vi "输入数据解析.vi"(0 "单个参数补充":dbl, 1 "从板号":dbl=1.0, 2 "主板二维码":string="BNET01", 3 "从板二维码":string="BNET01", 5 "主板引用":refnum<vi>, 7 "从板引用":refnum<vi>, 9 "主板选项":string="三级故障阀值", 11 "枚举":enum16{"主板", "从板"}(ring), 12 "快换":bool caption="快换写入") -> (4 "输出数组":dbl[][](array[numeric]), 6 "数组长度":dbl[](array[numeric]), 8 "循环次数":i32, 10 "命令":u32, 14 "名称":string[](array[string]), 15 "命令序号":u32[](array[numeric]))   [LabVIEW 2013] (continued)
                    n4439 = Unbundle By Name(w11573) -> ("总电压过低"=w11572:dbl)
                    n4440 = call "输入分辨率计算-EV05.vi"("1字节?"=FALSE, "数值"=w11572, "分辨率"=0.1) -> ("低字节"=w11575:dbl, "高字节1"=w11574:dbl)  [unwired: 2 in, 5 out]
                  }
                  frame Enabled {
                    w11578 = 255 ("高字节1")
                  }
                }
                n4441 = Build Array(w11570, w11571) -> (w11569:i32[])
              }
              frame 2 {
                # "温度过高"
                n4442 = disable-structure shown="启用" {
                  disable-tunnel: [w11585 255 ("高字节1")] -> w11581
                  disable-tunnel: w11579 -> [w11583 _]
                  frame Disabled {
                    n4443 = Unbundle By Name(w11583) -> ("温度过高"=w11582:dbl)
                    n4444 = call "输入分辨率计算-EV05.vi"("1字节?"=TRUE, "数值"=w11582, "偏移量"=-40.0, "分辨率"=1.0) -> ("高字节1"=w11585:dbl)  [unwired: 1 in, 6 out]
                  }
                  frame Enabled {
                  }
                }
                n4445 = Build Array(w11581) -> (w11580:i32[])
              }
              frame 3 {
                # "温度过低"
                n4446 = disable-structure shown="启用" {
                  disable-tunnel: [w11595 255 ("高字节1")] -> w11591
                  disable-tunnel: w11589 -> [w11593 _]
                  frame Disabled {
                    n4447 = Unbundle By Name(w11593) -> ("温度过低"=w11592:dbl)
                    n4448 = call "输入分辨率计算-EV05.vi"("1字节?"=TRUE, "数值"=w11592, "偏移量"=-40.0, "分辨率"=1.0) -> ("高字节1"=w11595:dbl)  [unwired: 1 in, 6 out]
                  }
                  frame Enabled {
                  }
                }
                n4449 = Build Array(w11591) -> (w11590:i32[])
              }
              frame 4 {
                # "整组温度不均衡"
                n4450 = disable-structure shown="启用" {
                  disable-tunnel: [w11605 255 ("高字节1")] -> w11601
                  disable-tunnel: w11599 -> [w11603 _]
                  frame Disabled {
                    n4451 = Unbundle By Name(w11603) -> ("整组温度不均衡"=w11602:dbl)
                    n4452 = call "输入分辨率计算-EV05.vi"("1字节?"=TRUE, "数值"=w11602, "偏移量"=0.0, "分辨率"=1.0) -> ("高字节1"=w11605:dbl)  [unwired: 1 in, 6 out]
                  }
                  frame Enabled {
                  }
                }
                n4453 = Build Array(w11601) -> (w11600:i32[])
              }
              frame 5 {
                # "单组电压不均衡"
                n4454 = disable-structure shown="启用" {
                  disable-tunnel: [w11617 w11620] -> w11612
                  disable-tunnel: [w11615 w11620] -> w11610
                  disable-tunnel: w11609 -> [w11614 _]
                  frame Disabled {
                    n4455 = Unbundle By Name(w11614) -> ("单组电压不均衡"=w11613:dbl)
                    n4456 = call "输入分辨率计算-EV05.vi"("1字节?"=FALSE, "数值"=w11613, "偏移量"=0.0, "分辨率"=0.001) -> ("低字节"=w11615:dbl, "高字节1"=w11617:dbl)  [unwired: 1 in, 5 out]
                  }
                  frame Enabled {
                    w11620 = 255 ("高字节1")
                  }
                }
                n4457 = Build Array(w11612, w11610) -> (w11611:i32[])
              }
              frame 6 {
                # "整组电压不均衡"
                n4458 = disable-structure shown="启用" {
                  disable-tunnel: [w11629 w11632] -> w11624
                  disable-tunnel: [w11627 w11632] -> w11622
                  disable-tunnel: w11621 -> [w11626 _]
                  frame Disabled {
                    n4459 = Unbundle By Name(w11626) -> ("整组电压不均衡"=w11625:dbl)
                    n4460 = call "输入分辨率计算-EV05.vi"("1字节?"=FALSE, "数值"=w11625, "偏移量"=0.0, "分辨率"=0.001) -> ("低字节"=w11627:dbl, "高字节1"=w11629:dbl)  [unwired: 1 in, 5 out]
                  }
                  frame Enabled {
                    w11632 = 255 ("高字节1")
                  }
                }
                n4461 = Build Array(w11624, w11622) -> (w11623:i32[])
              }
              frame 7 {
                # "单体电压过高"
                n4462 = disable-structure shown="启用" {
                  disable-tunnel: [w11641 w11644] -> w11636
                  disable-tunnel: [w11639 w11644] -> w11634
                  disable-tunnel: w11633 -> [w11638 _]
                  frame Disabled {
                    n4463 = Unbundle By Name(w11638) -> ("单体电压过高"=w11637:dbl)
                    n4464 = call "输入分辨率计算-EV05.vi"("1字节?"=FALSE, "数值"=w11637, "偏移量"=0.0, "分辨率"=0.001) -> ("低字节"=w11639:dbl, "高字节1"=w11641:dbl)  [unwired: 1 in, 5 out]
                  }
                  frame Enabled {
                    w11644 = 255 ("高字节1")
                  }
                }
                n4465 = Build Array(w11636, w11634) -> (w11635:i32[])
              }
              frame 8 {
                # "单体电压过低"
                n4466 = disable-structure shown="启用" {
                  disable-tunnel: [w11653 w11656] -> w11648
                  disable-tunnel: [w11651 w11656] -> w11646
                  disable-tunnel: w11645 -> [w11650 _]
                  frame Disabled {
                    n4467 = Unbundle By Name(w11650) -> ("单体电压过低"=w11649:dbl)
                    n4468 = call "输入分辨率计算-EV05.vi"("1字节?"=FALSE, "数值"=w11649, "偏移量"=0.0, "分辨率"=0.001) -> ("低字节"=w11651:dbl, "高字节1"=w11653:dbl)  [unwired: 1 in, 5 out]
                  }
                  frame Enabled {
                    w11656 = 255 ("高字节1")
                  }
                }
                n4469 = Build Array(w11648, w11646) -> (w11647:i32[])
              }
              frame 9 {
                # "充电电流过高"
                n4470 = disable-structure shown="启用" {
                  disable-tunnel: [w11665 w11668] -> w11660
                  disable-tunnel: [w11663 w11668] -> w11658
                  disable-tunnel: w11657 -> [w11662 _]
                  frame Disabled {
                    n4471 = Unbundle By Name(w11662) -> ("充电电流过高"=w11661:dbl)
                    n4472 = call "输入分辨率计算-EV05.vi"("1字节?"=FALSE, "数值"=w11661, "偏移量"=-3000.0, "分辨率"=0.1) -> ("低字节"=w11663:dbl, "高字节1"=w11665:dbl)  [unwired: 1 in, 5 out]
                  }
                  frame Enabled {
                    w11668 = 255 ("高字节1")
                  }
                }
                n4473 = Build Array(w11660, w11658) -> (w11659:i32[])
              }
              frame 10 {
                # "放电电流过高"
                n4474 = disable-structure shown="启用" {
                  disable-tunnel: [w11677 w11680] -> w11672
                  disable-tunnel: [w11675 w11680] -> w11670
                  disable-tunnel: w11669 -> [w11674 _]
                  frame Disabled {
                    n4475 = Unbundle By Name(w11674) -> ("放电电流过高"=w11673:dbl)
                    n4476 = call "输入分辨率计算-EV05.vi"("1字节?"=FALSE, "数值"=w11673, "偏移量"=-3000.0, "分辨率"=0.1) -> ("低字节"=w11675:dbl, "高字节1"=w11677:dbl)  [unwired: 1 in, 5 out]
                  }
                  frame Enabled {
                    w11680 = 255 ("高字节1")
                  }
                }
                n4477 = Build Array(w11672, w11670) -> (w11671:i32[])
              }
              frame 11 {
                # "单组温度不均衡"
                n4478 = disable-structure shown="启用" {
                  disable-tunnel: [w11687 255 ("高字节1")] -> w11683
                  disable-tunnel: w11681 -> [w11685 _]
                  frame Disabled {
                    n4479 = Unbundle By Name(w11685) -> ("单组温度不均衡"=w11684:dbl)
                    n4480 = call "输入分辨率计算-EV05.vi"("1字节?"=TRUE, "数值"=w11684, "偏移量"=0.0, "分辨率"=1.0) -> ("高字节1"=w11687:dbl)  [unwired: 1 in, 6 out]
                  }
                  frame Enabled {
                  }
                }
                n4481 = Build Array(w11683) -> (w11682:i32[])
              }
              frame 12 {
                # "SOC过高"
                n4482 = Unbundle By Name(w11694) -> ("SOC过高"=w11693:dbl)
                n4483 = call "输入分辨率计算-EV05.vi"("1字节?"=FALSE, "数值"=w11693, "偏移量"=0.0, "分辨率"=0.1) -> ("低字节"=w11691:dbl, "高字节1"=w11692:dbl)  [unwired: 1 in, 5 out]
                n4484 = Build Array(w11692, w11691) -> (w11696:dbl[])
              }
              frame 13 {
                # "SOC过低"
                n4485 = disable-structure shown="启用" {
                  disable-tunnel: w11701 -> [w11706 _]
                  disable-tunnel: [w11704 w11710] -> w11700
                  disable-tunnel: [w11703 w11710] -> w11699
                  frame Disabled {
                    n4486 = Unbundle By Name(w11706) -> ("SOC过低"=w11705:dbl)
                    n4487 = call "输入分辨率计算-EV05.vi"("1字节?"=FALSE, "数值"=w11705, "偏移量"=0.0, "分辨率"=0.1) -> ("低字节"=w11703:dbl, "高字节1"=w11704:dbl)  [unwired: 1 in, 5 out]
                  }
                  frame Enabled {
                    w11710 = 255 ("高字节1")
                  }
                }
                n4488 = Build Array(w11700, w11699) -> (w11702:i32[])
              }
              frame 14 {
                # "内阻过大"
                n4489 = disable-structure shown="启用" {
                  disable-tunnel: w11713 -> [w11718 _]
                  disable-tunnel: [w11714 255 ("高字节1")] -> w11711
                  frame Disabled {
                    n4490 = Unbundle By Name(w11718) -> ("内阻过大"=w11717:dbl)
                    n4491 = call "输入分辨率计算-EV05.vi"("1字节?"=TRUE, "数值"=w11717, "分辨率"=0.1) -> ("高字节1"=w11714:dbl)  [unwired: 2 in, 6 out]
                  }
                  frame Enabled {
                  }
                }
                n4492 = Build Array(w11711) -> (w11712:i32[])
              }
              frame 15 {
                # "极柱温度过高"
                n4493 = disable-structure shown="启用" {
                  disable-tunnel: w11722 -> [w11728 _]
                  disable-tunnel: [w11724 255 ("高字节1")] -> w11720
                  frame Disabled {
                    n4494 = Unbundle By Name(w11728) -> ("极柱温度过高"=w11727:dbl)
                    n4495 = call "输入分辨率计算-EV05.vi"("1字节?"=TRUE, "数值"=w11727, "偏移量"=-40.0, "分辨率"=1.0) -> ("高字节1"=w11724:dbl)  [unwired: 1 in, 6 out]
                  }
                  frame Enabled {
                  }
                }
                n4496 = Build Array(w11720) -> (w11721:i32[])
              }
              frame 16 {
                # "SOH过低"
                n4497 = disable-structure shown="启用" {
                  disable-tunnel: [w11745 w11753] -> w11732
                  disable-tunnel: w11731 -> [w11742 _]
                  disable-tunnel: [w11734 w11753] -> w11730
                  frame Disabled {
                    n4498 = Unbundle By Name(w11742) -> ("SOH过低"=w11741:dbl)
                    n4499 = call "输入分辨率计算-EV05.vi"("1字节?"=FALSE, "数值"=w11741, "偏移量"=0.0, "分辨率"=0.1) -> ("低字节"=w11743:dbl, "高字节1"=w11744:dbl)  [unwired: 1 in, 5 out]
                    n4500 = call "二进制解析-8.6.vi"("索引"=4, "数值"=w11744) -> ("低位子数组"=w11747:i32[])  [unwired: 3 out]
                    n4501 = call "二进制解析-8.6.vi"("索引"=4, "数值"=w11743) -> ("低位子数组"=w11736:i32[], "高位子数组"=w11746:i32[])  [unwired: 2 out]
                    n4502 = call "二进制解析-8.6.vi"("索引"=4, "数值"=0) -> ("低位子数组"=w11737:i32[])  [unwired: 3 out]
                    n4503 = Insert Into Array(array=w11747, new element=w11746) -> (w11740:i32[])  [unwired: 1 in]
                    n4504 = Insert Into Array(array=w11736, new element=w11737) -> (w11735:i32[])  [unwired: 1 in]
                    n4505 = call "数值二进制转十进制-8.6.vi"("子数组"=w11740) -> ("十进制数值"=w11745:i32)  [unwired: 4 out]
                    n4506 = call "数值二进制转十进制-8.6.vi"("子数组"=w11735) -> ("十进制数值"=w11734:i32)  [unwired: 4 out]
                  }
                  frame Enabled {
                    w11753 = 255 ("高字节1")
                  }
                }
                n4507 = Build Array(w11732, w11730) -> (w11733:i32[])
              }
            }
            n4508 = Insert Into Array(array=w11553, new element=w11554) -> (w11552:dbl[])  [unwired: 1 in]
          }
          n4509 = Build Array(w11549) -> (w11548:dbl[][])
          n4510 = Build Array("二级故障阀值") -> (w11539:string[])
        }
        frame "SOC过高(3)" {
          n4511 = Unbundle By Name(w11759) -> ("一级故障 3"=w11760:refnum<vi>)
          n4512 = property class="Clust (严格)"(reference=w11760) -> ("Value"=w11758:T4)  [unwired: 1 in, 2 out]
          n4513 = for {
            N: 17 -> [_]
            tunnel: w11758 -> [w11770]
            shift-right: [w11767] -> w11764
            shift-left: dbl[] [] -> [w11768]
            i -> [w11771]
            n4514 = case shown="12" w11771 {
              tunnel: w11770 -> [w11772 w11783 w11794 w11804 w11814 w11824 w11836 w11848 w11860 w11872 w11884 w11896 w11909 w11917 w11924 w11933 w11942]
              tunnel: [w11773 w11784 w11795 w11805 w11815 w11826 w11838 w11850 w11862 w11874 w11886 w11897 w11911 w11919 w11923 w11932 w11944] -> w11769
              frame 0, Default {
                # "总电压过高"
                n4515 = disable-structure shown="启用" {
                  disable-tunnel: [w11779 w11782] -> w11775
                  disable-tunnel: [w11778 w11782] -> w11774
                  disable-tunnel: w11772 -> [w11777 _]
                  frame Disabled {
                    n4516 = Unbundle By Name(w11777) -> ("总电压过高"=w11776:dbl)
                    n4517 = call "输入分辨率计算-EV05.vi"("1字节?"=FALSE, "数值"=w11776, "分辨率"=0.1) -> ("低字节"=w11779:dbl, "高字节1"=w11778:dbl)  [unwired: 2 in, 5 out]
                  }
                  frame Enabled {
                    w11782 = 255 ("高字节1")
                  }
                }
                n4518 = Build Array(w11774, w11775) -> (w11773:i32[])
              }
              frame 1 {
                # "总电压过低"
                n4519 = disable-structure shown="启用" {
                  disable-tunnel: [w11790 w11793] -> w11786
                  disable-tunnel: [w11789 w11793] -> w11785
                  disable-tunnel: w11783 -> [w11788 _]
                  frame Disabled {
                    n4520 = Unbundle By Name(w11788) -> ("总电压过低"=w11787:dbl)
                    n4521 = call "输入分辨率计算-EV05.vi"("1字节?"=FALSE, "数值"=w11787, "分辨率"=0.1) -> ("低字节"=w11790:dbl, "高字节1"=w11789:dbl)  [unwired: 2 in, 5 out]
                  }
                  frame Enabled {
                    w11793 = 255 ("高字节1")
                  }
                }
                n4522 = Build Array(w11785, w11786) -> (w11784:i32[])
              }
              frame 2 {
                # "温度过高"
                n4523 = disable-structure shown="启用" {
                  disable-tunnel: [w11800 255 ("高字节1")] -> w11796
                  disable-tunnel: w11794 -> [w11798 _]
                  frame Disabled {
                    n4524 = Unbundle By Name(w11798) -> ("温度过高"=w11797:dbl)
                    n4525 = call "输入分辨率计算-EV05.vi"("1字节?"=TRUE, "数值"=w11797, "偏移量"=-40.0, "分辨率"=1.0) -> ("高字节1"=w11800:dbl)  [unwired: 1 in, 6 out]
                  }
                  frame Enabled {
                  }
                }
                n4526 = Build Array(w11796) -> (w11795:i32[])
              }
              frame 3 {
                # "温度过低"
                n4527 = disable-structure shown="启用" {
                  disable-tunnel: [w11810 255 ("高字节1")] -> w11806
                  disable-tunnel: w11804 -> [w11808 _]
                  frame Disabled {
                    n4528 = Unbundle By Name(w11808) -> ("温度过低"=w11807:dbl)
                    n4529 = call "输入分辨率计算-EV05.vi"("1字节?"=TRUE, "数值"=w11807, "偏移量"=-40.0, "分辨率"=1.0) -> ("高字节1"=w11810:dbl)  [unwired: 1 in, 6 out]
                  }
                  frame Enabled {
                  }
                }
                n4530 = Build Array(w11806) -> (w11805:i32[])
              }
              frame 4 {
                # "整组温度不均衡"
                n4531 = disable-structure shown="启用" {
                  disable-tunnel: [w11820 255 ("高字节1")] -> w11816
                  disable-tunnel: w11814 -> [w11818 _]
                  frame Disabled {
                    n4532 = Unbundle By Name(w11818) -> ("整组温度不均衡"=w11817:dbl)
                    n4533 = call "输入分辨率计算-EV05.vi"("1字节?"=TRUE, "数值"=w11817, "偏移量"=0.0, "分辨率"=1.0) -> ("高字节1"=w11820:dbl)  [unwired: 1 in, 6 out]
                  }
                  frame Enabled {
                  }
                }
                n4534 = Build Array(w11816) -> (w11815:i32[])
              }
              frame 5 {
                # "单组电压不均衡"
                n4535 = disable-structure shown="启用" {
                  disable-tunnel: [w11832 w11835] -> w11827
                  disable-tunnel: [w11830 w11835] -> w11825
                  disable-tunnel: w11824 -> [w11829 _]
                  frame Disabled {
                    n4536 = Unbundle By Name(w11829) -> ("单组电压不均衡"=w11828:dbl)
                    n4537 = call "输入分辨率计算-EV05.vi"("1字节?"=FALSE, "数值"=w11828, "偏移量"=0.0, "分辨率"=0.001) -> ("低字节"=w11830:dbl, "高字节1"=w11832:dbl)  [unwired: 1 in, 5 out]
                  }
                  frame Enabled {
                    w11835 = 255 ("高字节1")
                  }
                }
                n4538 = Build Array(w11827, w11825) -> (w11826:i32[])
              }
              frame 6 {
                # "整组电压不均衡"
                n4539 = disable-structure shown="启用" {
                  disable-tunnel: [w11844 w11847] -> w11839
                  disable-tunnel: [w11842 w11847] -> w11837
                  disable-tunnel: w11836 -> [w11841 _]
                  frame Disabled {
                    n4540 = Unbundle By Name(w11841) -> ("整组电压不均衡"=w11840:dbl)
                    n4541 = call "输入分辨率计算-EV05.vi"("1字节?"=FALSE, "数值"=w11840, "偏移量"=0.0, "分辨率"=0.001) -> ("低字节"=w11842:dbl, "高字节1"=w11844:dbl)  [unwired: 1 in, 5 out]
                  }
                  frame Enabled {
                    w11847 = 255 ("高字节1")
                  }
                }
                n4542 = Build Array(w11839, w11837) -> (w11838:i32[])
              }
              frame 7 {
                # "单体电压过高"
                n4543 = disable-structure shown="启用" {
                  disable-tunnel: [w11856 w11859] -> w11851
                  disable-tunnel: [w11854 w11859] -> w11849
                  disable-tunnel: w11848 -> [w11853 _]
                  frame Disabled {
                    n4544 = Unbundle By Name(w11853) -> ("单体电压过高"=w11852:dbl)
                    n4545 = call "输入分辨率计算-EV05.vi"("1字节?"=FALSE, "数值"=w11852, "偏移量"=0.0, "分辨率"=0.001) -> ("低字节"=w11854:dbl, "高字节1"=w11856:dbl)  [unwired: 1 in, 5 out]
                  }
                  frame Enabled {
                    w11859 = 255 ("高字节1")
                  }
                }
                n4546 = Build Array(w11851, w11849) -> (w11850:i32[])
              }
              frame 8 {
                # "单体电压过低"
                n4547 = disable-structure shown="启用" {
                  disable-tunnel: [w11868 w11871] -> w11863
                  disable-tunnel: [w11866 w11871] -> w11861
                  disable-tunnel: w11860 -> [w11865 _]
                  frame Disabled {
                    n4548 = Unbundle By Name(w11865) -> ("单体电压过低"=w11864:dbl)
                    n4549 = call "输入分辨率计算-EV05.vi"("1字节?"=FALSE, "数值"=w11864, "偏移量"=0.0, "分辨率"=0.001) -> ("低字节"=w11866:dbl, "高字节1"=w11868:dbl)  [unwired: 1 in, 5 out]
                  }
                  frame Enabled {
                    w11871 = 255 ("高字节1")
                  }
                }
                n4550 = Build Array(w11863, w11861) -> (w11862:i32[])
              }
              frame 9 {
                # "充电电流过高"
                n4551 = disable-structure shown="启用" {
                  disable-tunnel: [w11880 w11883] -> w11875
                  disable-tunnel: [w11878 w11883] -> w11873
                  disable-tunnel: w11872 -> [w11877 _]
                  frame Disabled {
                    n4552 = Unbundle By Name(w11877) -> ("充电电流过高"=w11876:dbl)
                    n4553 = call "输入分辨率计算-EV05.vi"("1字节?"=FALSE, "数值"=w11876, "偏移量"=-3000.0, "分辨率"=0.1) -> ("低字节"=w11878:dbl, "高字节1"=w11880:dbl)  [unwired: 1 in, 5 out]
                  }
                  frame Enabled {
                    w11883 = 255 ("高字节1")
                  }
                }
                n4554 = Build Array(w11875, w11873) -> (w11874:i32[])
              }
              frame 10 {
                # "放电电流过高"
                n4555 = disable-structure shown="启用" {
                  disable-tunnel: [w11892 w11895] -> w11887
                  disable-tunnel: [w11890 w11895] -> w11885
                  disable-tunnel: w11884 -> [w11889 _]
                  frame Disabled {
                    n4556 = Unbundle By Name(w11889) -> ("放电电流过高"=w11888:dbl)
                    n4557 = call "输入分辨率计算-EV05.vi"("1字节?"=FALSE, "数值"=w11888, "偏移量"=-3000.0, "分辨率"=0.1) -> ("低字节"=w11890:dbl, "高字节1"=w11892:dbl)  [unwired: 1 in, 5 out]
                  }
                  frame Enabled {
                    w11895 = 255 ("高字节1")
                  }
                }
                n4558 = Build Array(w11887, w11885) -> (w11886:i32[])
              }
              frame 11 {
                # "单组温度不均衡"
                n4559 = disable-structure shown="启用" {
                  disable-tunnel: [w11902 255 ("高字节1")] -> w11898
                  disable-tunnel: w11896 -> [w11900 _]
                  frame Disabled {
                    n4560 = Unbundle By Name(w11900) -> ("单组温度不均衡"=w11899:dbl)
                    n4561 = call "输入分辨率计算-EV05.vi"("1字节?"=TRUE, "数值"=w11899, "偏移量"=0.0, "分辨率"=1.0) -> ("高字节1"=w11902:dbl)  [unwired: 1 in, 6 out]
                  }
                  frame Enabled {
                  }
                }
                n4562 = Build Array(w11898) -> (w11897:i32[])
              }
              frame 12 {
                # "SOC过高"
                n4563 = Unbundle By Name(w11909) -> ("SOC过高"=w11908:dbl)
                n4564 = call "输入分辨率计算-EV05.vi"("1字节?"=FALSE, "数值"=w11908, "偏移量"=0.0, "分辨率"=0.1) -> ("低字节"=w11906:dbl, "高字节1"=w11907:dbl)  [unwired: 1 in, 5 out]
                n4565 = Build Array(w11907, w11906) -> (w11911:dbl[])
              }
              frame 13 {
                # "SOC过低"
                n4566 = Unbundle By Name(w11917) -> ("SOC过低"=w11916:dbl)
                n4567 = call "输入分辨率计算-EV05.vi"("1字节?"=FALSE, "数值"=w11916, "偏移量"=0.0, "分辨率"=0.1) -> ("低字节"=w11914:dbl, "高字节1"=w11915:dbl)  [unwired: 1 in, 5 out]
                n4568 = Build Array(w11915, w11914) -> (w11919:dbl[])
              }
              frame 14 {
                # "内阻过大"
                n4569 = disable-structure shown="启用" {
                  disable-tunnel: w11924 -> [w11929 _]
                  disable-tunnel: [w11925 255 ("高字节1")] -> w11922
                  frame Disabled {
                    n4570 = Unbundle By Name(w11929) -> ("内阻过大"=w11928:dbl)
                    n4571 = call "输入分辨率计算-EV05.vi"("1字节?"=TRUE, "数值"=w11928, "分辨率"=0.1) -> ("高字节1"=w11925:dbl)  [unwired: 2 in, 6 out]
                  }
                  frame Enabled {
                  }
                }
                n4572 = Build Array(w11922) -> (w11923:i32[])
              }
              frame 15 {
                # "极柱温度过高"
                n4573 = disable-structure shown="启用" {
                  disable-tunnel: w11933 -> [w11939 _]
                  disable-tunnel: [w11935 255 ("高字节1")] -> w11931
                  frame Disabled {
                    n4574 = Unbundle By Name(w11939) -> ("极柱温度过高"=w11938:dbl)
                    n4575 = call "输入分辨率计算-EV05.vi"("1字节?"=TRUE, "数值"=w11938, "偏移量"=-40.0, "分辨率"=1.0) -> ("高字节1"=w11935:dbl)  [unwired: 1 in, 6 out]
                  }
                  frame Enabled {
                  }
                }
                n4576 = Build Array(w11931) -> (w11932:i32[])
              }
              frame 16 {
                # "SOH过低"
                n4577 = disable-structure shown="启用" {
                  disable-tunnel: [w11956 w11964] -> w11943
                  disable-tunnel: w11942 -> [w11953 _]
                  disable-tunnel: [w11945 w11964] -> w11941
                  frame Disabled {
                    n4578 = Unbundle By Name(w11953) -> ("SOH过低"=w11952:dbl)
                    n4579 = call "输入分辨率计算-EV05.vi"("1字节?"=FALSE, "数值"=w11952, "偏移量"=0.0, "分辨率"=0.1) -> ("低字节"=w11954:dbl, "高字节1"=w11955:dbl)  [unwired: 1 in, 5 out]
                    n4580 = call "二进制解析-8.6.vi"("索引"=4, "数值"=w11955) -> ("低位子数组"=w11958:i32[])  [unwired: 3 out]
                    n4581 = call "二进制解析-8.6.vi"("索引"=4, "数值"=w11954) -> ("低位子数组"=w11947:i32[], "高位子数组"=w11957:i32[])  [unwired: 2 out]
                    n4582 = call "二进制解析-8.6.vi"("索引"=4, "数值"=0) -> ("低位子数组"=w11948:i32[])  [unwired: 3 out]
                    n4583 = Insert Into Array(array=w11958, new element=w11957) -> (w11951:i32[])  [unwired: 1 in]
                    n4584 = Insert Into Array(array=w11947, new element=w11948) -> (w11946:i32[])  [unwired: 1 in]
                    n4585 = call "数值二进制转十进制-8.6.vi"("子数组"=w11951) -> ("十进制数值"=w11956:i32)  [unwired: 4 out]
                    n4586 = call "数值二进制转十进制-8.6.vi"("子数组"=w11946) -> ("十进制数值"=w11945:i32)  [unwired: 4 out]
                  }
                  frame Enabled {
                    w11964 = 255 ("高字节1")
                  }
                }
                n4587 = Build Array(w11943, w11941) -> (w11944:i32[])
              }
            }
            n4588 = Insert Into Array(array=w11768, new element=w11769) -> (w11767:dbl[])  [unwired: 1 in]
          }
          n4589 = Build Array(w11764) -> (w11763:dbl[][])
          n4590 = Build Array("三级故障阀值") -> (w11754:string[])
        }
        frame "SOC过低" {
          n4591 = Unbundle By Name(w11970) -> ("一级故障"=w11971:refnum<vi>)
          n4592 = property class="Clust (严格)"(reference=w11971) -> ("Value"=w11969:T4)  [unwired: 1 in, 2 out]
          n4593 = for {
            N: 17 -> [_]
            tunnel: w11969 -> [w11981]
            shift-right: [w11978] -> w11975
            shift-left: dbl[] [] -> [w11979]
            i -> [w11982]
            n4594 = case shown="12" w11982 {
              tunnel: w11981 -> [w11983 w11994 w12005 w12015 w12025 w12035 w12047 w12059 w12071 w12083 w12095 w12107 w12119 w12131 w12138 w12147 w12156]
              tunnel: [w11984 w11995 w12006 w12016 w12026 w12037 w12049 w12061 w12073 w12085 w12097 w12108 w12121 w12133 w12137 w12146 w12158] -> w11980
              frame 0, Default {
                # "总电压过高"
                n4595 = disable-structure shown="启用" {
                  disable-tunnel: [w11990 w11993] -> w11986
                  disable-tunnel: [w11989 w11993] -> w11985
                  disable-tunnel: w11983 -> [w11988 _]
                  frame Disabled {
                    n4596 = Unbundle By Name(w11988) -> ("总电压过高"=w11987:dbl)
                    n4597 = call "输入分辨率计算-EV05.vi"("1字节?"=FALSE, "数值"=w11987, "分辨率"=0.1) -> ("低字节"=w11990:dbl, "高字节1"=w11989:dbl)  [unwired: 2 in, 5 out]
                  }
                  frame Enabled {
                    w11993 = 255 ("高字节1")
                  }
                }
                n4598 = Build Array(w11985, w11986) -> (w11984:i32[])
              }
              frame 1 {
                # "总电压过低"
                n4599 = disable-structure shown="启用" {
                  disable-tunnel: [w12001 w12004] -> w11997
                  disable-tunnel: [w12000 w12004] -> w11996
                  disable-tunnel: w11994 -> [w11999 _]
                  frame Disabled {
                    n4600 = Unbundle By Name(w11999) -> ("总电压过低"=w11998:dbl)
                    n4601 = call "输入分辨率计算-EV05.vi"("1字节?"=FALSE, "数值"=w11998, "分辨率"=0.1) -> ("低字节"=w12001:dbl, "高字节1"=w12000:dbl)  [unwired: 2 in, 5 out]
                  }
                  frame Enabled {
                    w12004 = 255 ("高字节1")
                  }
                }
                n4602 = Build Array(w11996, w11997) -> (w11995:i32[])
              }
              frame 2 {
                # "温度过高"
                n4603 = disable-structure shown="启用" {
                  disable-tunnel: [w12011 255 ("高字节1")] -> w12007
                  disable-tunnel: w12005 -> [w12009 _]
                  frame Disabled {
                    n4604 = Unbundle By Name(w12009) -> ("温度过高"=w12008:dbl)
                    n4605 = call "输入分辨率计算-EV05.vi"("1字节?"=TRUE, "数值"=w12008, "偏移量"=-40.0, "分辨率"=1.0) -> ("高字节1"=w12011:dbl)  [unwired: 1 in, 6 out]
                  }
                  frame Enabled {
                  }
                }
                n4606 = Build Array(w12007) -> (w12006:i32[])
              }
              frame 3 {
                # "温度过低"
                n4607 = disable-structure shown="启用" {
                  disable-tunnel: [w12021 255 ("高字节1")] -> w12017
                  disable-tunnel: w12015 -> [w12019 _]
                  frame Disabled {
                    n4608 = Unbundle By Name(w12019) -> ("温度过低"=w12018:dbl)
                    n4609 = call "输入分辨率计算-EV05.vi"("1字节?"=TRUE, "数值"=w12018, "偏移量"=-40.0, "分辨率"=1.0) -> ("高字节1"=w12021:dbl)  [unwired: 1 in, 6 out]
                  }
                  frame Enabled {
                  }
                }
                n4610 = Build Array(w12017) -> (w12016:i32[])
              }
              frame 4 {
                # "整组温度不均衡"
                n4611 = disable-structure shown="启用" {
                  disable-tunnel: [w12031 255 ("高字节1")] -> w12027
                  disable-tunnel: w12025 -> [w12029 _]
                  frame Disabled {
                    n4612 = Unbundle By Name(w12029) -> ("整组温度不均衡"=w12028:dbl)
                    n4613 = call "输入分辨率计算-EV05.vi"("1字节?"=TRUE, "数值"=w12028, "偏移量"=0.0, "分辨率"=1.0) -> ("高字节1"=w12031:dbl)  [unwired: 1 in, 6 out]
                  }
                  frame Enabled {
                  }
                }
                n4614 = Build Array(w12027) -> (w12026:i32[])
              }
              frame 5 {
                # "单组电压不均衡"
                n4615 = disable-structure shown="启用" {
                  disable-tunnel: [w12043 w12046] -> w12038
                  disable-tunnel: [w12041 w12046] -> w12036
                  disable-tunnel: w12035 -> [w12040 _]
                  frame Disabled {
                    n4616 = Unbundle By Name(w12040) -> ("单组电压不均衡"=w12039:dbl)
                    n4617 = call "输入分辨率计算-EV05.vi"("1字节?"=FALSE, "数值"=w12039, "偏移量"=0.0, "分辨率"=0.001) -> ("低字节"=w12041:dbl, "高字节1"=w12043:dbl)  [unwired: 1 in, 5 out]
                  }
                  frame Enabled {
                    w12046 = 255 ("高字节1")
                  }
                }
                n4618 = Build Array(w12038, w12036) -> (w12037:i32[])
              }
              frame 6 {
                # "整组电压不均衡"
                n4619 = disable-structure shown="启用" {
                  disable-tunnel: [w12055 w12058] -> w12050
                  disable-tunnel: [w12053 w12058] -> w12048
                  disable-tunnel: w12047 -> [w12052 _]
                  frame Disabled {
                    n4620 = Unbundle By Name(w12052) -> ("整组电压不均衡"=w12051:dbl)
                    n4621 = call "输入分辨率计算-EV05.vi"("1字节?"=FALSE, "数值"=w12051, "偏移量"=0.0, "分辨率"=0.001) -> ("低字节"=w12053:dbl, "高字节1"=w12055:dbl)  [unwired: 1 in, 5 out]
                  }
                  frame Enabled {
                    w12058 = 255 ("高字节1")
                  }
                }
                n4622 = Build Array(w12050, w12048) -> (w12049:i32[])
              }
              frame 7 {
                # "单体电压过高"
                n4623 = disable-structure shown="启用" {
                  disable-tunnel: [w12067 w12070] -> w12062
                  disable-tunnel: [w12065 w12070] -> w12060
                  disable-tunnel: w12059 -> [w12064 _]
                  frame Disabled {
                    n4624 = Unbundle By Name(w12064) -> ("单体电压过高"=w12063:dbl)
                    n4625 = call "输入分辨率计算-EV05.vi"("1字节?"=FALSE, "数值"=w12063, "偏移量"=0.0, "分辨率"=0.001) -> ("低字节"=w12065:dbl, "高字节1"=w12067:dbl)  [unwired: 1 in, 5 out]
                  }
                  frame Enabled {
                    w12070 = 255 ("高字节1")
                  }
                }
                n4626 = Build Array(w12062, w12060) -> (w12061:i32[])
              }
              frame 8 {
                # "单体电压过低"
                n4627 = disable-structure shown="启用" {
                  disable-tunnel: [w12079 w12082] -> w12074
                  disable-tunnel: [w12077 w12082] -> w12072
                  disable-tunnel: w12071 -> [w12076 _]
                  frame Disabled {
                    n4628 = Unbundle By Name(w12076) -> ("单体电压过低"=w12075:dbl)
                    n4629 = call "输入分辨率计算-EV05.vi"("1字节?"=FALSE, "数值"=w12075, "偏移量"=0.0, "分辨率"=0.001) -> ("低字节"=w12077:dbl, "高字节1"=w12079:dbl)  [unwired: 1 in, 5 out]
                  }
                  frame Enabled {
                    w12082 = 255 ("高字节1")
                  }
                }
                n4630 = Build Array(w12074, w12072) -> (w12073:i32[])
              }
              frame 9 {
                # "充电电流过高"
                n4631 = disable-structure shown="启用" {
                  disable-tunnel: [w12091 w12094] -> w12086
                  disable-tunnel: [w12089 w12094] -> w12084
                  disable-tunnel: w12083 -> [w12088 _]
                  frame Disabled {
                    n4632 = Unbundle By Name(w12088) -> ("充电电流过高"=w12087:dbl)
                    n4633 = call "输入分辨率计算-EV05.vi"("1字节?"=FALSE, "数值"=w12087, "偏移量"=-3000.0, "分辨率"=0.1) -> ("低字节"=w12089:dbl, "高字节1"=w12091:dbl)  [unwired: 1 in, 5 out]
                  }
                  frame Enabled {
                    w12094 = 255 ("高字节1")
                  }
                }
                n4634 = Build Array(w12086, w12084) -> (w12085:i32[])
              }
              frame 10 {
                # "放电电流过高"
                n4635 = disable-structure shown="启用" {
                  disable-tunnel: [w12103 w12106] -> w12098
                  disable-tunnel: [w12101 w12106] -> w12096
                  disable-tunnel: w12095 -> [w12100 _]
                  frame Disabled {
                    n4636 = Unbundle By Name(w12100) -> ("放电电流过高"=w12099:dbl)
                    n4637 = call "输入分辨率计算-EV05.vi"("1字节?"=FALSE, "数值"=w12099, "偏移量"=-3000.0, "分辨率"=0.1) -> ("低字节"=w12101:dbl, "高字节1"=w12103:dbl)  [unwired: 1 in, 5 out]
                  }
                  frame Enabled {
                    w12106 = 255 ("高字节1")
                  }
                }
                n4638 = Build Array(w12098, w12096) -> (w12097:i32[])
              }
              frame 11 {
                # "单组温度不均衡"
                n4639 = disable-structure shown="启用" {
                  disable-tunnel: [w12113 255 ("高字节1")] -> w12109
                  disable-tunnel: w12107 -> [w12111 _]
                  frame Disabled {
                    n4640 = Unbundle By Name(w12111) -> ("单组温度不均衡"=w12110:dbl)
                    n4641 = call "输入分辨率计算-EV05.vi"("1字节?"=TRUE, "数值"=w12110, "偏移量"=0.0, "分辨率"=1.0) -> ("高字节1"=w12113:dbl)  [unwired: 1 in, 6 out]
                  }
                  frame Enabled {
                  }
                }
                n4642 = Build Array(w12109) -> (w12108:i32[])
              }
              frame 12 {
                # "SOC过高"
                n4643 = Unbundle By Name(w12119) -> ("SOC过高"=w12118:dbl)
                n4644 = call "输入分辨率计算-EV05.vi"("1字节?"=FALSE, "数值"=w12118, "偏移量"=0.0, "分辨率"=0.1) -> ()  [unwired: 1 in, 7 out]
                n4645 = disable-structure shown="启用" {
                  disable-tunnel: _ -> [w12125 _]
                  disable-tunnel: [w12125 255 ("高字节1")] -> w12117
                  disable-tunnel: [w12124 i32[] [] ("低位子数组")] -> _
                  disable-tunnel: _ -> [w12124 _]
                  frame Disabled {
                  }
                  frame Enabled {
                  }
                }
                n4646 = Build Array(w12117, w12117) -> (w12121:i32[])
              }
              frame 13 {
                # "SOC过低"
                n4647 = Unbundle By Name(w12131) -> ("SOC过低"=w12130:dbl)
                n4648 = call "输入分辨率计算-EV05.vi"("1字节?"=FALSE, "数值"=w12130, "偏移量"=0.0, "分辨率"=0.1) -> ("低字节"=w12128:dbl, "高字节1"=w12129:dbl)  [unwired: 1 in, 5 out]
                n4649 = Build Array(w12129, w12128) -> (w12133:dbl[])
              }
              frame 14 {
                # "内阻过大"
                n4650 = disable-structure shown="启用" {
                  disable-tunnel: w12138 -> [w12143 _]
                  disable-tunnel: [w12139 255 ("高字节1")] -> w12136
                  frame Disabled {
                    n4651 = Unbundle By Name(w12143) -> ("内阻过大"=w12142:dbl)
                    n4652 = call "输入分辨率计算-EV05.vi"("1字节?"=TRUE, "数值"=w12142, "分辨率"=0.1) -> ("高字节1"=w12139:dbl)  [unwired: 2 in, 6 out]
                  }
                  frame Enabled {
                  }
                }
                n4653 = Build Array(w12136) -> (w12137:i32[])
              }
              frame 15 {
                # "极柱温度过高"
                n4654 = disable-structure shown="启用" {
                  disable-tunnel: w12147 -> [w12153 _]
                  disable-tunnel: [w12149 255 ("高字节1")] -> w12145
                  frame Disabled {
                    n4655 = Unbundle By Name(w12153) -> ("极柱温度过高"=w12152:dbl)
                    n4656 = call "输入分辨率计算-EV05.vi"("1字节?"=TRUE, "数值"=w12152, "偏移量"=-40.0, "分辨率"=1.0) -> ("高字节1"=w12149:dbl)  [unwired: 1 in, 6 out]
                  }
                  frame Enabled {
                  }
                }
                n4657 = Build Array(w12145) -> (w12146:i32[])
              }
              frame 16 {
                # "SOH过低"
                n4658 = disable-structure shown="启用" {
                  disable-tunnel: [w12170 w12178] -> w12157
                  disable-tunnel: w12156 -> [w12167 _]
                  disable-tunnel: [w12159 w12178] -> w12155
                  frame Disabled {
                    n4659 = Unbundle By Name(w12167) -> ("SOH过低"=w12166:dbl)
                    n4660 = call "输入分辨率计算-EV05.vi"("1字节?"=FALSE, "数值"=w12166, "偏移量"=0.0, "分辨率"=0.1) -> ("低字节"=w12168:dbl, "高字节1"=w12169:dbl)  [unwired: 1 in, 5 out]
                    n4661 = call "二进制解析-8.6.vi"("索引"=4, "数值"=w12169) -> ("低位子数组"=w12172:i32[])  [unwired: 3 out]
                    n4662 = call "二进制解析-8.6.vi"("索引"=4, "数值"=w12168) -> ("低位子数组"=w12161:i32[], "高位子数组"=w12171:i32[])  [unwired: 2 out]
                    n4663 = call "二进制解析-8.6.vi"("索引"=4, "数值"=0) -> ("低位子数组"=w12162:i32[])  [unwired: 3 out]
                    n4664 = Insert Into Array(array=w12172, new element=w12171) -> (w12165:i32[])  [unwired: 1 in]
                    n4665 = Insert Into Array(array=w12161, new element=w12162) -> (w12160:i32[])  [unwired: 1 in]
                    n4666 = call "数值二进制转十进制-8.6.vi"("子数组"=w12165) -> ("十进制数值"=w12170:i32)  [unwired: 4 out]
                    n4667 = call "数值二进制转十进制-8.6.vi"("子数组"=w12160) -> ("十进制数值"=w12159:i32)  [unwired: 4 out]
                  }
                  frame Enabled {
                    w12178 = 255 ("高字节1")
                  }
                }
                n4668 = Build Array(w12157, w12155) -> (w12158:i32[])
              }
            }
            n4669 = Insert Into Array(array=w11979, new element=w11980) -> (w11978:dbl[])  [unwired: 1 in]
          }
          n4670 = Build Array(w11975) -> (w11974:dbl[][])
          n4671 = Build Array("一级故障阀值") -> (w11965:string[])
        }
        frame "SOC过低(2)" {
          n4672 = Unbundle By Name(w12184) -> ("一级故障 2"=w12185:refnum<vi>)
          n4673 = property class="Clust (严格)"(reference=w12185) -> ("Value"=w12183:T4)  [unwired: 1 in, 2 out]
          n4674 = for {
            N: 17 -> [_]
            tunnel: w12183 -> [w12195]
            shift-right: [w12192] -> w12189
            shift-left: dbl[] [] -> [w12193]
            i -> [w12196]
            n4675 = case shown="12" w12196 {
              tunnel: w12195 -> [w12197 w12208 w12219 w12229 w12239 w12249 w12261 w12273 w12285 w12297 w12309 w12321 w12333 w12345 w12352 w12361 w12370]
              tunnel: [w12198 w12209 w12220 w12230 w12240 w12251 w12263 w12275 w12287 w12299 w12311 w12322 w12335 w12347 w12351 w12360 w12372] -> w12194
              frame 0, Default {
                # "总电压过高"
                n4676 = disable-structure shown="启用" {
                  disable-tunnel: [w12204 w12207] -> w12200
                  disable-tunnel: [w12203 w12207] -> w12199
                  disable-tunnel: w12197 -> [w12202 _]
                  frame Disabled {
                    n4677 = Unbundle By Name(w12202) -> ("总电压过高"=w12201:dbl)
                    n4678 = call "输入分辨率计算-EV05.vi"("1字节?"=FALSE, "数值"=w12201, "分辨率"=0.1) -> ("低字节"=w12204:dbl, "高字节1"=w12203:dbl)  [unwired: 2 in, 5 out]
                  }
                  frame Enabled {
                    w12207 = 255 ("高字节1")
                  }
                }
                n4679 = Build Array(w12199, w12200) -> (w12198:i32[])
              }
              frame 1 {
                # "总电压过低"
                n4680 = disable-structure shown="启用" {
                  disable-tunnel: [w12215 w12218] -> w12211
                  disable-tunnel: [w12214 w12218] -> w12210
                  disable-tunnel: w12208 -> [w12213 _]
                  frame Disabled {
                    n4681 = Unbundle By Name(w12213) -> ("总电压过低"=w12212:dbl)
                    n4682 = call "输入分辨率计算-EV05.vi"("1字节?"=FALSE, "数值"=w12212, "分辨率"=0.1) -> ("低字节"=w12215:dbl, "高字节1"=w12214:dbl)  [unwired: 2 in, 5 out]
                  }
                  frame Enabled {
                    w12218 = 255 ("高字节1")
                  }
                }
                n4683 = Build Array(w12210, w12211) -> (w12209:i32[])
              }
              frame 2 {
                # "温度过高"
                n4684 = disable-structure shown="启用" {
                  disable-tunnel: [w12225 255 ("高字节1")] -> w12221
                  disable-tunnel: w12219 -> [w12223 _]
                  frame Disabled {
                    n4685 = Unbundle By Name(w12223) -> ("温度过高"=w12222:dbl)
                    n4686 = call "输入分辨率计算-EV05.vi"("1字节?"=TRUE, "数值"=w12222, "偏移量"=-40.0, "分辨率"=1.0) -> ("高字节1"=w12225:dbl)  [unwired: 1 in, 6 out]
                  }
                  frame Enabled {
                  }
                }
                n4687 = Build Array(w12221) -> (w12220:i32[])
              }
              frame 3 {
                # "温度过低"
                n4688 = disable-structure shown="启用" {
                  disable-tunnel: [w12235 255 ("高字节1")] -> w12231
                  disable-tunnel: w12229 -> [w12233 _]
                  frame Disabled {
                    n4689 = Unbundle By Name(w12233) -> ("温度过低"=w12232:dbl)
                    n4690 = call "输入分辨率计算-EV05.vi"("1字节?"=TRUE, "数值"=w12232, "偏移量"=-40.0, "分辨率"=1.0) -> ("高字节1"=w12235:dbl)  [unwired: 1 in, 6 out]
                  }
                  frame Enabled {
                  }
                }
                n4691 = Build Array(w12231) -> (w12230:i32[])
              }
              frame 4 {
                # "整组温度不均衡"
                n4692 = disable-structure shown="启用" {
                  disable-tunnel: [w12245 255 ("高字节1")] -> w12241
                  disable-tunnel: w12239 -> [w12243 _]
                  frame Disabled {
                    n4693 = Unbundle By Name(w12243) -> ("整组温度不均衡"=w12242:dbl)
                    n4694 = call "输入分辨率计算-EV05.vi"("1字节?"=TRUE, "数值"=w12242, "偏移量"=0.0, "分辨率"=1.0) -> ("高字节1"=w12245:dbl)  [unwired: 1 in, 6 out]
                  }
                  frame Enabled {
                  }
                }
                n4695 = Build Array(w12241) -> (w12240:i32[])
              }
              frame 5 {
                # "单组电压不均衡"
                n4696 = disable-structure shown="启用" {
                  disable-tunnel: [w12257 w12260] -> w12252
                  disable-tunnel: [w12255 w12260] -> w12250
                  disable-tunnel: w12249 -> [w12254 _]
                  frame Disabled {
                    n4697 = Unbundle By Name(w12254) -> ("单组电压不均衡"=w12253:dbl)
                    n4698 = call "输入分辨率计算-EV05.vi"("1字节?"=FALSE, "数值"=w12253, "偏移量"=0.0, "分辨率"=0.001) -> ("低字节"=w12255:dbl, "高字节1"=w12257:dbl)  [unwired: 1 in, 5 out]
                  }
                  frame Enabled {
                    w12260 = 255 ("高字节1")
                  }
                }
                n4699 = Build Array(w12252, w12250) -> (w12251:i32[])
              }
              frame 6 {
                # "整组电压不均衡"
                n4700 = disable-structure shown="启用" {
                  disable-tunnel: [w12269 w12272] -> w12264
                  disable-tunnel: [w12267 w12272] -> w12262
                  disable-tunnel: w12261 -> [w12266 _]
                  frame Disabled {
                    n4701 = Unbundle By Name(w12266) -> ("整组电压不均衡"=w12265:dbl)
                    n4702 = call "输入分辨率计算-EV05.vi"("1字节?"=FALSE, "数值"=w12265, "偏移量"=0.0, "分辨率"=0.001) -> ("低字节"=w12267:dbl, "高字节1"=w12269:dbl)  [unwired: 1 in, 5 out]
                  }
                  frame Enabled {
                    w12272 = 255 ("高字节1")
                  }
                }
                n4703 = Build Array(w12264, w12262) -> (w12263:i32[])
              }
              frame 7 {
                # "单体电压过高"
                n4704 = disable-structure shown="启用" {
                  disable-tunnel: [w12281 w12284] -> w12276
                  disable-tunnel: [w12279 w12284] -> w12274
                  disable-tunnel: w12273 -> [w12278 _]
                  frame Disabled {
                    n4705 = Unbundle By Name(w12278) -> ("单体电压过高"=w12277:dbl)
                    n4706 = call "输入分辨率计算-EV05.vi"("1字节?"=FALSE, "数值"=w12277, "偏移量"=0.0, "分辨率"=0.001) -> ("低字节"=w12279:dbl, "高字节1"=w12281:dbl)  [unwired: 1 in, 5 out]
                  }
                  frame Enabled {
                    w12284 = 255 ("高字节1")
                  }
                }
                n4707 = Build Array(w12276, w12274) -> (w12275:i32[])
              }
              frame 8 {
                # "单体电压过低"
                n4708 = disable-structure shown="启用" {
                  disable-tunnel: [w12293 w12296] -> w12288
                  disable-tunnel: [w12291 w12296] -> w12286
                  disable-tunnel: w12285 -> [w12290 _]
                  frame Disabled {
                    n4709 = Unbundle By Name(w12290) -> ("单体电压过低"=w12289:dbl)
                    n4710 = call "输入分辨率计算-EV05.vi"("1字节?"=FALSE, "数值"=w12289, "偏移量"=0.0, "分辨率"=0.001) -> ("低字节"=w12291:dbl, "高字节1"=w12293:dbl)  [unwired: 1 in, 5 out]
                  }
                  frame Enabled {
                    w12296 = 255 ("高字节1")
                  }
                }
                n4711 = Build Array(w12288, w12286) -> (w12287:i32[])
              }
              frame 9 {
                # "充电电流过高"
                n4712 = disable-structure shown="启用" {
                  disable-tunnel: [w12305 w12308] -> w12300
                  disable-tunnel: [w12303 w12308] -> w12298
                  disable-tunnel: w12297 -> [w12302 _]
                  frame Disabled {
                    n4713 = Unbundle By Name(w12302) -> ("充电电流过高"=w12301:dbl)
                    n4714 = call "输入分辨率计算-EV05.vi"("1字节?"=FALSE, "数值"=w12301, "偏移量"=-3000.0, "分辨率"=0.1) -> ("低字节"=w12303:dbl, "高字节1"=w12305:dbl)  [unwired: 1 in, 5 out]
                  }
                  frame Enabled {
                    w12308 = 255 ("高字节1")
                  }
                }
                n4715 = Build Array(w12300, w12298) -> (w12299:i32[])
              }
              frame 10 {
                # "放电电流过高"
                n4716 = disable-structure shown="启用" {
                  disable-tunnel: [w12317 w12320] -> w12312
                  disable-tunnel: [w12315 w12320] -> w12310
                  disable-tunnel: w12309 -> [w12314 _]
                  frame Disabled {
                    n4717 = Unbundle By Name(w12314) -> ("放电电流过高"=w12313:dbl)
                    n4718 = call "输入分辨率计算-EV05.vi"("1字节?"=FALSE, "数值"=w12313, "偏移量"=-3000.0, "分辨率"=0.1) -> ("低字节"=w12315:dbl, "高字节1"=w12317:dbl)  [unwired: 1 in, 5 out]
                  }
                  frame Enabled {
                    w12320 = 255 ("高字节1")
                  }
                }
                n4719 = Build Array(w12312, w12310) -> (w12311:i32[])
              }
              frame 11 {
                # "单组温度不均衡"
                n4720 = disable-structure shown="启用" {
                  disable-tunnel: [w12327 255 ("高字节1")] -> w12323
                  disable-tunnel: w12321 -> [w12325 _]
                  frame Disabled {
                    n4721 = Unbundle By Name(w12325) -> ("单组温度不均衡"=w12324:dbl)
                    n4722 = call "输入分辨率计算-EV05.vi"("1字节?"=TRUE, "数值"=w12324, "偏移量"=0.0, "分辨率"=1.0) -> ("高字节1"=w12327:dbl)  [unwired: 1 in, 6 out]
                  }
                  frame Enabled {
                  }
                }
                n4723 = Build Array(w12323) -> (w12322:i32[])
              }
              frame 12 {
                # "SOC过高"
                n4724 = Unbundle By Name(w12333) -> ("SOC过高"=w12332:dbl)
                n4725 = call "输入分辨率计算-EV05.vi"("1字节?"=FALSE, "数值"=w12332, "偏移量"=0.0, "分辨率"=0.1) -> ()  [unwired: 1 in, 7 out]
                n4726 = disable-structure shown="启用" {
                  disable-tunnel: _ -> [w12339 _]
                  disable-tunnel: [w12339 255 ("高字节1")] -> w12331
                  disable-tunnel: [w12338 i32[] [] ("低位子数组")] -> _
                  disable-tunnel: _ -> [w12338 _]
                  frame Disabled {
                  }
                  frame Enabled {
                  }
                }
                n4727 = Build Array(w12331, w12331) -> (w12335:i32[])
              }
              frame 13 {
                # "SOC过低"
                n4728 = Unbundle By Name(w12345) -> ("SOC过低"=w12344:dbl)
                n4729 = call "输入分辨率计算-EV05.vi"("1字节?"=FALSE, "数值"=w12344, "偏移量"=0.0, "分辨率"=0.1) -> ("低字节"=w12342:dbl, "高字节1"=w12343:dbl)  [unwired: 1 in, 5 out]
                n4730 = Build Array(w12343, w12342) -> (w12347:dbl[])
              }
              frame 14 {
                # "内阻过大"
                n4731 = disable-structure shown="启用" {
                  disable-tunnel: w12352 -> [w12357 _]
                  disable-tunnel: [w12353 255 ("高字节1")] -> w12350
                  frame Disabled {
                    n4732 = Unbundle By Name(w12357) -> ("内阻过大"=w12356:dbl)
                    n4733 = call "输入分辨率计算-EV05.vi"("1字节?"=TRUE, "数值"=w12356, "分辨率"=0.1) -> ("高字节1"=w12353:dbl)  [unwired: 2 in, 6 out]
                  }
                  frame Enabled {
                  }
                }
                n4734 = Build Array(w12350) -> (w12351:i32[])
              }
              frame 15 {
                # "极柱温度过高"
                n4735 = disable-structure shown="启用" {
                  disable-tunnel: w12361 -> [w12367 _]
                  disable-tunnel: [w12363 255 ("高字节1")] -> w12359
                  frame Disabled {
                    n4736 = Unbundle By Name(w12367) -> ("极柱温度过高"=w12366:dbl)
                    n4737 = call "输入分辨率计算-EV05.vi"("1字节?"=TRUE, "数值"=w12366, "偏移量"=-40.0, "分辨率"=1.0) -> ("高字节1"=w12363:dbl)  [unwired: 1 in, 6 out]
                  }
                  frame Enabled {
                  }
                }
                n4738 = Build Array(w12359) -> (w12360:i32[])
              }
              frame 16 {
                # "SOH过低"
                n4739 = disable-structure shown="启用" {
                  disable-tunnel: [w12384 w12392] -> w12371
                  disable-tunnel: w12370 -> [w12381 _]
                  disable-tunnel: [w12373 w12392] -> w12369
                  frame Disabled {
                    n4740 = Unbundle By Name(w12381) -> ("SOH过低"=w12380:dbl)
                    n4741 = call "输入分辨率计算-EV05.vi"("1字节?"=FALSE, "数值"=w12380, "偏移量"=0.0, "分辨率"=0.1) -> ("低字节"=w12382:dbl, "高字节1"=w12383:dbl)  [unwired: 1 in, 5 out]
                    n4742 = call "二进制解析-8.6.vi"("索引"=4, "数值"=w12383) -> ("低位子数组"=w12386:i32[])  [unwired: 3 out]
                    n4743 = call "二进制解析-8.6.vi"("索引"=4, "数值"=w12382) -> ("低位子数组"=w12375:i32[], "高位子数组"=w12385:i32[])  [unwired: 2 out]
                    n4744 = call "二进制解析-8.6.vi"("索引"=4, "数值"=0) -> ("低位子数组"=w12376:i32[])  [unwired: 3 out]
                    n4745 = Insert Into Array(array=w12386, new element=w12385) -> (w12379:i32[])  [unwired: 1 in]
                    n4746 = Insert Into Array(array=w12375, new element=w12376) -> (w12374:i32[])  [unwired: 1 in]
                    n4747 = call "数值二进制转十进制-8.6.vi"("子数组"=w12379) -> ("十进制数值"=w12384:i32)  [unwired: 4 out]
                    n4748 = call "数值二进制转十进制-8.6.vi"("子数组"=w12374) -> ("十进制数值"=w12373:i32)  [unwired: 4 out]
                  }
                  frame Enabled {
                    w12392 = 255 ("高字节1")
                  }
